vi "Data entry form.vi"(0 "Stack in":refnum<class "Stack.lvclass">, 5 "Position":dbl, 7 "Module Type":string, 9 "Module?":bool, 11 "error in (no error)":errorcluster, 12 "Operator":string) -> (4 "Stack out":refnum<class "Stack.lvclass">, 15 "error out":errorcluster)   [LabVIEW 2021, in "Stack.lvclass"]
uses:
  Stack.lvclass
  Stack.lvclass/Stack.ctl
panel:
  out "Sensor thickness":string
  out "BP Type":string
  out "Geometry":string
  in  "Proto thickness for glue dispense":dbl
  out "Resolution":string
  out "Date":string
  in  "Glue Batch":string
  in  "Component Tray ID":string
  in  "Assembly Tray ID":string
  in  "PUT ID":string
  in  "Baselayer ID":string
  in  "Toplayer ID":string
  in  "Submit":bool
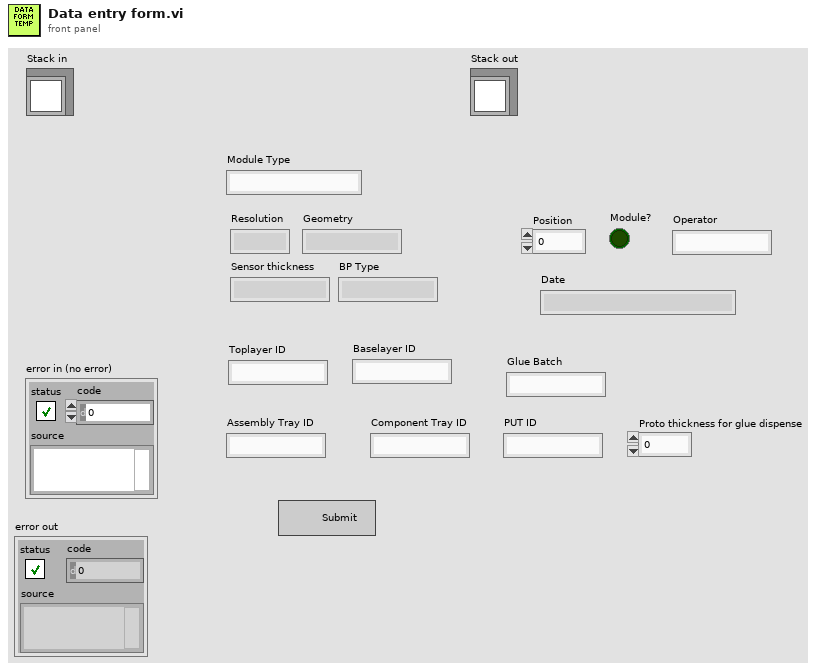
[diagram p1: front panel]
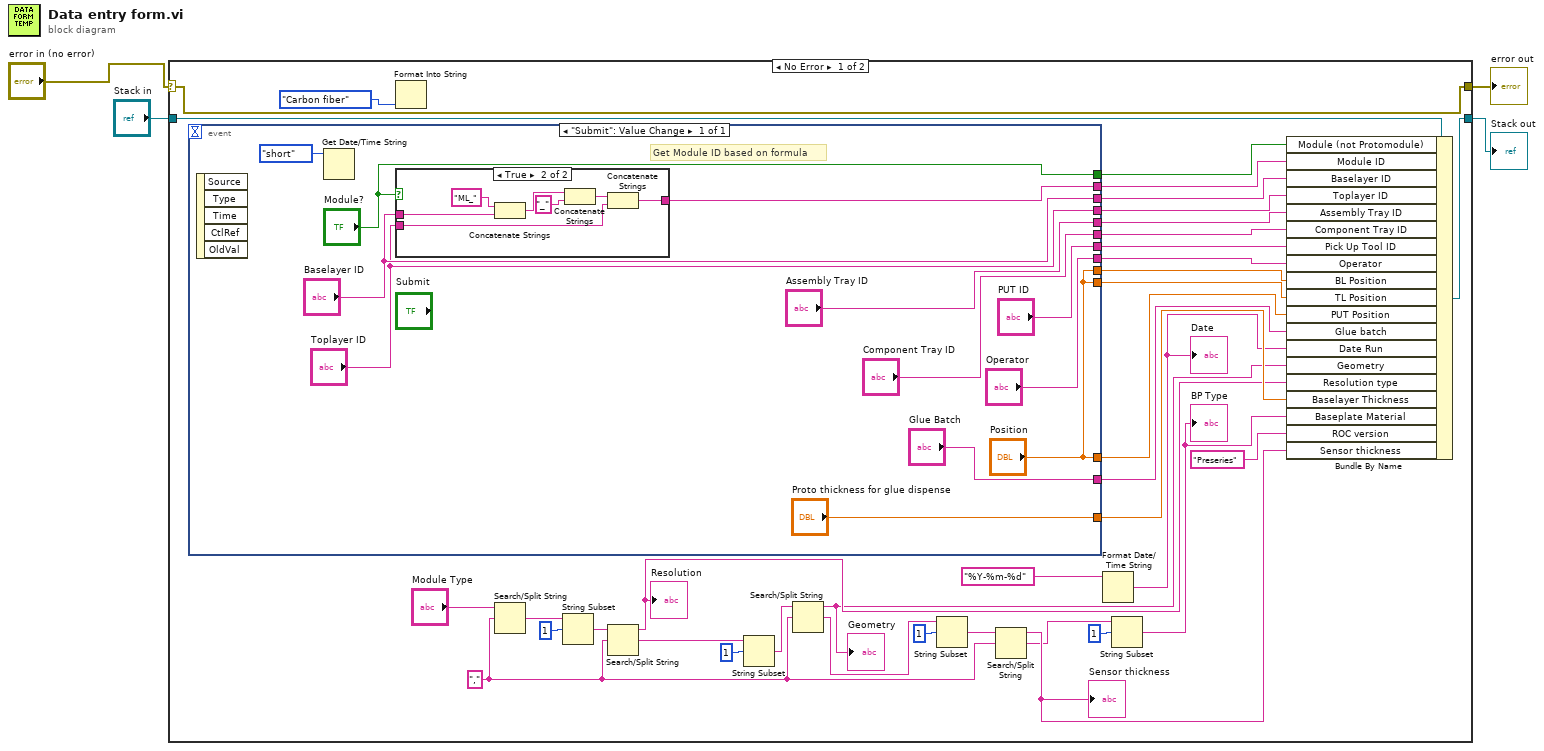
[diagram p0: block diagram]
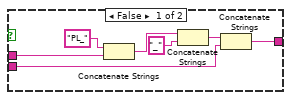
[diagram p2: hidden frame]
diagram:
  n1 = case shown="No Error" "error in (no error)" {
    selector: "error in (no error)" -> [w41 w69]
    tunnel: [w41 w69] -> w3
    tunnel: [w40 w68] -> w1
    tunnel: "Stack in" -> [w27 w68]
    frame No Error {
      w10 = "," ("search string/char (-)")
      n2 = event shown="[0] \"Submit\": Value Change" {
        selector: _ -> [_]
        dyn-events: _ -> [_]
        timeout: _ -> [_]
        tunnel: ["Toplayer ID"] -> w39
        tunnel: ["Baselayer ID"] -> w38
        tunnel: ["Component Tray ID"] -> w37
        tunnel: ["Assembly Tray ID"] -> w36
        tunnel: ["PUT ID"] -> w35
        tunnel: ["Operator"] -> w34
        tunnel: ["Module?"] -> w33
        tunnel: ["Position"] -> w32
        tunnel: ["Position"] -> w31
        tunnel: ["Position"] -> w30
        tunnel: [w46] -> w29
        tunnel: ["Glue Batch"] -> w28
        tunnel: ["Proto thickness for glue dispense"] -> w26
        event "Submit": Value Change {
          # "Get Module ID based on formula"
          n3 = event-data() -> ()  [unwired: 1 in, 5 out]
          n4 = Get Date/Time String(date format (0)=enum16{"short", "long", "abbreviated"}."short") -> ()  [unwired: 2 in, 2 out]
          n5 = case shown="True" "Module?" {
            tunnel: "Baselayer ID" -> [w56 w63]
            tunnel: "Toplayer ID" -> [w55 w65]
            tunnel: [w54 w64] -> w46
            frame False {
              n6 = Concatenate Strings("PL_" ("string"), w56) -> (w60:string)
              n7 = Concatenate Strings(w60, "_" ("string")) -> (w59:string)
              n8 = Concatenate Strings(w59, w55) -> (w54:string)
            }
            frame True {
              n9 = Concatenate Strings("ML_" ("string"), w63) -> (w62:string)
              n10 = Concatenate Strings(w62, "_" ("string")) -> (w66:string)
              n11 = Concatenate Strings(w66, w65) -> (w64:string)
            }
          }
        }
      }
      n12 = Format Into String(enum16{"CuW", "PCB", "Carbon fiber"}."Carbon fiber") -> ()  [unwired: 3 in, 2 out]
      n13 = Search/Split String(string="Module Type", search string/char (-)=w10) -> (match + rest of string=w19:string)  [unwired: 1 in, 2 out]
      n14 = String Subset(string=w19, offset (0)=1) -> (substring=w18:string)  [unwired: 1 in]
      n15 = Search/Split String(string=w18, search string/char (-)=w10) -> (substring before match=w14:string, match + rest of string=w16:string)  [unwired: 1 in, 1 out]
      "Resolution" <- w14
      n16 = String Subset(string=w16, offset (0)=1) -> (substring=w15:string)  [unwired: 1 in]
      n17 = Search/Split String(string=w15, search string/char (-)=w10) -> (substring before match=w11:string, match + rest of string=w6:string)  [unwired: 1 in, 1 out]
      "Geometry" <- w11
      n18 = String Subset(string=w6, offset (0)=1) -> (substring=w12:string)  [unwired: 1 in]
      n19 = Search/Split String(string=w12, search string/char (-)=w10) -> (substring before match=w9:string, match + rest of string=w5:string)  [unwired: 1 in, 1 out]
      "Sensor thickness" <- w9
      n20 = Format Date/Time String(time format string (%c)="%Y-%m-%d") -> (date/time string=w24:string)  [unwired: 2 in]
      "Date" <- w24
      n21 = String Subset(string=w5, offset (0)=1) -> (substring=w7:string)  [unwired: 1 in]
      "BP Type" <- w7
      n22 = Bundle By Name(cluster=w27, "Module (not Protomodule)"=w33, "Module ID"=w29, "Baselayer ID"=w38, "Toplayer ID"=w39, "Assembly Tray ID"=w36, "Component Tray ID"=w37, "Pick Up Tool ID"=w35, "Operator"=w34, "BL Position"=w32, "TL Position"=w31, "PUT Position"=w30, "Glue batch"=w28, "Date Run"=w24, "Geometry"=w11, "Resolution type"=w14, "Baselayer Thickness"=w26, "Baseplate Material"=w7, "ROC version"="Preseries", "Sensor thickness"=w9) -> (w40:refnum<class "Stack.lvclass">)
    }
    frame Error {
    }
  }
  "error out" <- w3
  "Stack out" <- w1
